vi "main.vi"() -> ()   [LabVIEW 2015]
uses:
  <vilib>/Platform/TimedLoop/XDataNode/timing_clust.ctl
  <vilib>/Platform/TimedLoop/XDataNode/nitl_modes.ctl
  <vilib>/Platform/TimedLoop/XDataNode/wakeup.ctl
  <vilib>/rvi/Emulation/niFpgaSctlEmulationGetInTimedLoop.vi
  <vilib>/rvi/Emulation/niFpgaEmulationReportErrorSimple.vi
  <vilib>/rvi/Emulation/niFpgaGetClockAttributes.vi
  <vilib>/rvi/Emulation/niFpgaCriticalErrorInLSC.vi
  <vilib>/rvi/eio/common/nirviEmuTemplateMethod_errors.vi
  <vilib>/Platform/TimedLoop/XDataNode/XDataNode.xnode
  <vilib>/eio/EIOMethodNode/EIOMethodNode.xnode
  <vilib>/eio/EIONode/EIONode.xnode
  <vilib>/Platform/TimedLoop/XDataNode/XDNodeRunTimeDep.lvlib
panel:
  out "RAM_OUT":u8
  in  "ram_adress":u16
  in  "ram_data":u8
  in  "we":bool
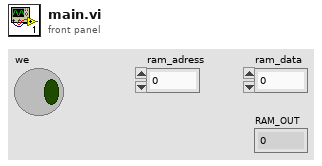
[diagram p1: front panel]
types:
  T1 = typedef "XDNodeRunTimeDep.lvlib/timing_clust.ctl" = cluster{"Expected End [f-1]":u64, "Actual End [f-1]":u64, "Finished Late? [f-1]":bool, "Expected End [i-1]":u64, "Actual End [i-1]":u64, "Finished Late? [i-1]":bool, "Expected Start [i]":u64, "Actual Start [i]":u64, "Expected Start [f]":u64, "Actual Start [f]":u64, "Source Name":string, "Structure Name":string, "Period":i64, "Deadline":i64, "Offset":i64, "Start":i64, "Priority":i32, "Timeout":i32, "Mode":T2, "Wakeup Reason":T3, "Error":errorcluster, "Source Type":string, "Secondary Source Type":string, "Global End Time":u64, "Global Start Time":u64, "Frame Duration":u64, "Iteration Duration":u64, "Assigned CPU":i32, "I/O Scan Engine Mode":u32}
  T2 = typedef "XDNodeRunTimeDep.lvlib/nitl_modes.ctl" = enum32{"No Change", "Process missed periods, maintain original phase", "Discard missed periods, maintain original phase", "Process missed periods, ignore original phase", "Discard missed periods, ignore original phase"}
  T3 = typedef "XDNodeRunTimeDep.lvlib/wakeup.ctl" = enum32{"Normal", "Aborted", "Asynchronous wakeup", "Timing source error", "Timed loop error", "Timeout"}
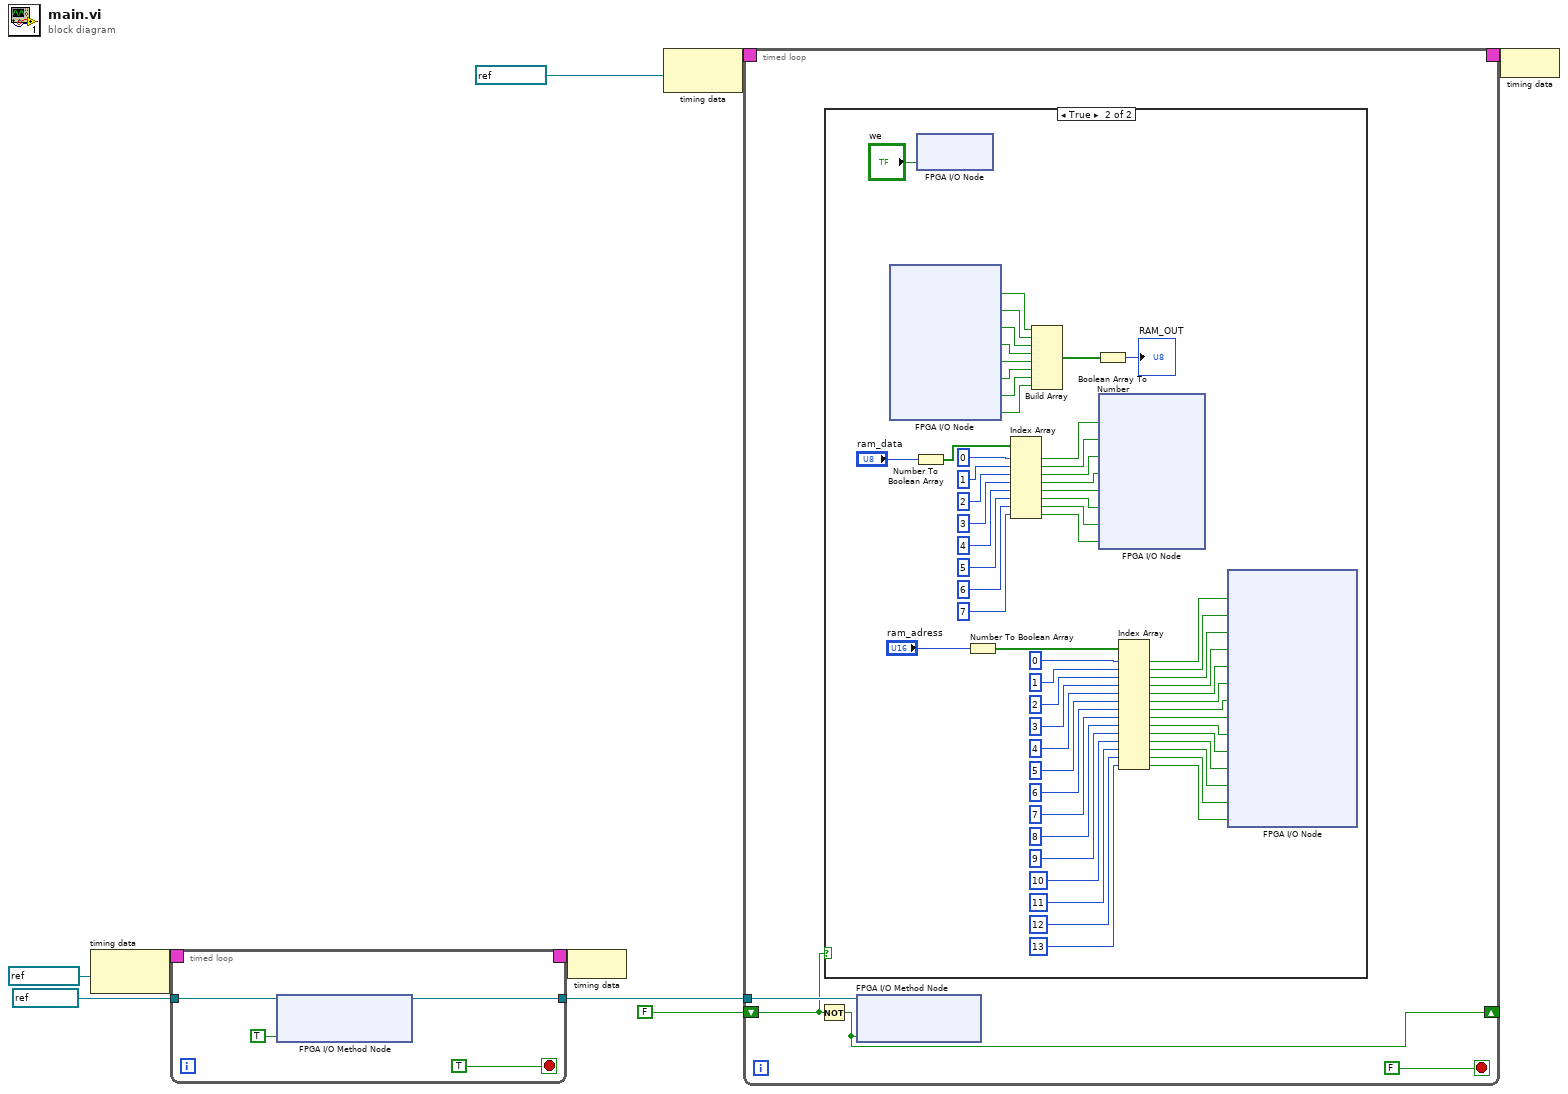
[diagram p0: block diagram]
diagram:
  n1 = node-c288(refnum<k21> "100MHz" ("Source Name")) -> (w6:T1)
  n2 = timed-loop {
    timing: w6 -> [_]
    timing-out: [_] -> w5
    tunnel: refnum<k21> "inpCLK" ("FPGA I/O In") -> [w13]
    tunnel: [w10] -> w2
    stop <- TRUE stop-if-true
    n3 = xnode "FPGA I/O Method Node"("FPGA I/O In"=w13, "Enable"=TRUE) -> ("FPGA I/O Out"=w10:refnum<k21>)
  }
  n4 = node-c288(w5) -> ()
  n5 = node-c288(refnum<k21> "100MHz" ("Source Name")) -> (w9:T1)
  n6 = timed-loop {
    timing: w9 -> [_]
    timing-out: [_] -> w8
    tunnel: w2 -> [w19]
    shift-right: [w17] -> _
    shift-left: FALSE -> [w16]
    stop <- FALSE stop-if-true
    n7 = Not(x=w16) -> (.not. x?=w17:bool)
    n8 = case shown="True" w16 {
      frame False {
      }
      frame True {
        n9 = xnode "FPGA I/O Node"() -> ("RAM_OUT[0]"=w29:bool, "RAM_OUT[1]"=w28:bool, "RAM_OUT[2]"=w27:bool, "RAM_OUT[3]"=w24:bool, "RAM_OUT[4]"=w23:bool, "RAM_OUT[5]"=w22:bool, "RAM_OUT[6]"=w20:bool, "RAM_OUT[7]"=w21:bool)  [unwired: 8 in, 8 out]
        n10 = Number To Boolean Array(number="ram_data") -> (Boolean array=w77:bool[])
        n11 = xnode "FPGA I/O Node"("we"="we") -> ()  [unwired: 1 in, 1 out]
        n12 = Number To Boolean Array(number="ram_adress") -> (Boolean array=w59:bool[])
        n13 = Index Array(array=w77, index #1=0 ("index"), index #2=1 ("index"), index #3=2 ("index"), index #4=3 ("index"), index #5=4 ("index"), index #6=5 ("index"), index #7=6 ("index"), index #8=7 ("index")) -> (element #1=w76:bool, element #2=w75:bool, element #3=w74:bool, element #4=w73:bool, element #5=w72:bool, element #6=w71:bool, element #7=w70:bool, element #8=w69:bool)
        n14 = Build Array(w29, w28, w27, w24, w23, w22, w20, w21) -> (w25:bool[])
        n15 = Boolean Array To Number(Boolean array=w25) -> (number=→"RAM_OUT":u8)
        n16 = xnode "FPGA I/O Node"("ram_data[0]"=w76, "ram_data[1]"=w75, "ram_data[2]"=w74, "ram_data[3]"=w73, "ram_data[4]"=w72, "ram_data[5]"=w71, "ram_data[6]"=w70, "ram_data[7]"=w69) -> ()  [unwired: 8 in, 8 out]
        n17 = Index Array(array=w59, index #1=0 ("index"), index #2=1 ("index"), index #3=2 ("index"), index #4=3 ("index"), index #5=4 ("index"), index #6=5 ("index"), index #7=6 ("index"), index #8=7 ("index"), index #9=8 ("index"), index #10=9 ("index"), index #11=10 ("index"), index #12=11 ("index"), index #13=12 ("index"), index #14=13 ("index")) -> (element #1=w49:bool, element #2=w48:bool, element #3=w47:bool, element #4=w46:bool, element #5=w45:bool, element #6=w44:bool, element #7=w43:bool, element #8=w42:bool, element #9=w41:bool, element #10=w40:bool, element #11=w39:bool, element #12=w38:bool, element #13=w37:bool, element #14=w36:bool)
        n18 = xnode "FPGA I/O Node"("ram_address[0]"=w49, "ram_address[1]"=w48, "ram_address[2]"=w47, "ram_address[3]"=w46, "ram_address[4]"=w45, "ram_address[5]"=w44, "ram_address[6]"=w43, "ram_address[7]"=w42, "ram_address[8]"=w41, "ram_address[9]"=w40, "ram_address[10]"=w39, "ram_address[11]"=w38, "ram_address[12]"=w37, "ram_address[13]"=w36) -> ()  [unwired: 14 in, 14 out]
      }
    }
    n19 = xnode "FPGA I/O Method Node"("FPGA I/O In"=w19, "Data"=w17) -> ()  [unwired: 1 out]
  }
  n20 = node-c288(w8) -> ()
